vi "Meas Result Add Reading.vi"(6 "reading":T3, 8 "error in":errorcluster, 9 "f [Hz]":dbl, 10 "fid":i32, 11 "results ref":refnum<vi>) -> (0 "error out":errorcluster, 3 "result data":T1)   [LabVIEW 2013]
doc: "Adds single reading to the result."
uses:
  Meas Results.ctl
  bridge/Bridge Frequency Readings Data.ctl
  bridge/Bridge Reading Data.ctl
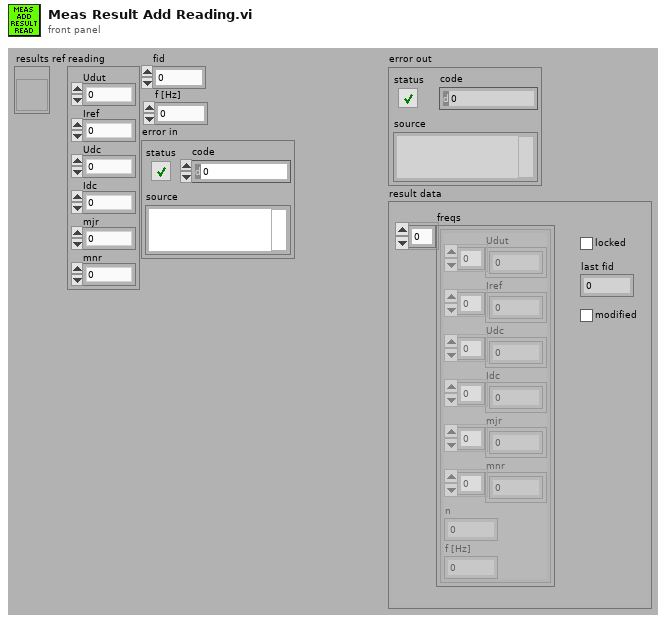
[diagram p1: front panel]
types:
  T1 = typedef "Meas Results.ctl" = cluster{"freqs":T2[], "locked":bool, "last fid":i32, "modified":bool}
  T2 = typedef "Bridge Frequency Readings Data.ctl" = cluster{"Udut":dbl[], "Iref":dbl[], "Udc":dbl[], "Idc":dbl[], "mjr":dbl[], "mnr":dbl[], "n":i32, "f [Hz]":dbl}
  T3 = typedef "Bridge Reading Data.ctl" = cluster{"Udut":dbl, "Iref":dbl, "Udc":dbl, "Idc":dbl, "mjr":dbl, "mnr":dbl}
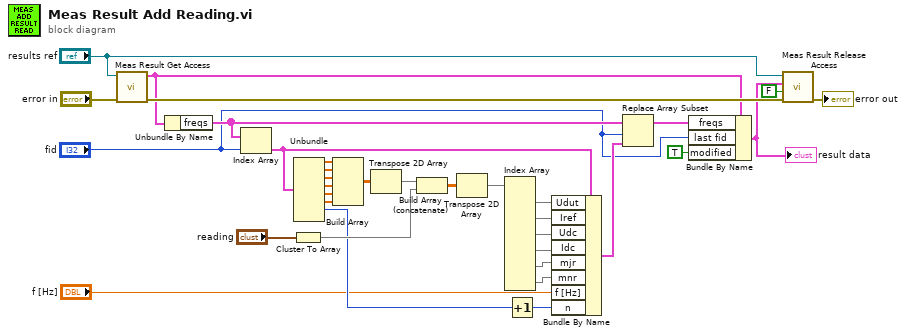
[diagram p0: block diagram]
diagram:
  n1 = call "Meas Result Get Access.vi"("error in"="error in", "results ref"="results ref") -> ("error out"=w14:errorcluster, "results data"=w12:T1)  [unwired: 8 in]
  n2 = Unbundle By Name(w12) -> ("freqs"=w15:T2[])
  n3 = Index Array(array=w15, index="fid") -> (element=w25:T2)
  n4 = Cluster To Array(cluster="reading") -> (array=w27:dbl[])
  n5 = Unbundle(w25) -> ("Udut"=w34:dbl[], "Iref"=w33:dbl[], "Udc"=w32:dbl[], "Idc"=w31:dbl[], "mjr"=w30:dbl[], "mnr"=w29:dbl[], "n"=w17:i32)  [unwired: 1 out]
  n6 = Build Array(w34, w33, w32, w31, w30, w29) -> (w28:dbl[][])
  n7 = Transpose 2D Array(2D array=w28) -> (transposed array=w2:dbl[][])
  n8 = Build Array (concatenate)(w2, w27) -> (w26:dbl[][])
  n9 = Transpose 2D Array(2D array=w26) -> (transposed array=w1:dbl[][])
  n10 = Index Array(array=w1) -> (element #1=w24:dbl[], element #2=w23:dbl[], element #3=w22:dbl[], element #4=w21:dbl[], element #5=w20:dbl[], element #6=w19:dbl[])  [unwired: 12 in]
  n11 = Increment(x=w17) -> (x+1=w18:i32)
  n12 = Bundle By Name(cluster=w25, "Udut"=w24, "Iref"=w23, "Udc"=w22, "Idc"=w21, "mjr"=w20, "mnr"=w19, "f [Hz]"="f [Hz]", "n"=w18) -> (w16:T2)
  n13 = Replace Array Subset(array=w15, new element=w16, index="fid") -> (w13:T2[])
  n14 = Bundle By Name(cluster=w12, "freqs"=w13, "last fid"="fid", "modified"=TRUE) -> (w11:T1)
  "result data" <- w11
  n15 = call "Meas Result Release Access.vi"("error in"=w14, "Release only (True)"=FALSE, "results data in"=w11, "results ref"="results ref") -> ("error out"=→"error out":errorcluster)  [unwired: 7 in]
